vi "Configure Write LabVIEW Measurement File.vi"(0 "subVI":refnum<vi>, 2 "VI":refnum<vi>, 3 "ParentVI":refnum<vi>) -> (1 "Data Valid":bool)   [LabVIEW 2020]
doc: "Writes data to text-based measurement files (.lvm), binary measurement files (.tdm or .tdms), or Microsoft Excel files (.xlsx)."
uses:
  <vilib>/express/express shared/ExFile.llb/ex_FileFormats.ctl
  <vilib>/express/express shared/ExFile.llb/ex_userDefProperty.ctl
  <vilib>/express/express shared/ex_EditUserDefinedProperties/usiDataType.ctl
  <vilib>/express/express shared/ExFile.llb/ex_propertySource.ctl
  <vilib>/express/express output/ExFileWriteBlock.llb/ex_ExcelAdvancedConfig.ctl
  <vilib>/express/express shared/ExFile.llb/ex_FileGlobals.vi
  <vilib>/express/express shared/NI_ExcelFile/NI_ExcelFile.lvlib
panel:
  in  "timestamp":T1={"absolute time"=TRUE, "Timestamp format"=""}
  in  "Configure User Def Prop In":T5
  in  "Advanced":bool
  in  "Streaming":bool
  in  "always hostless warning":string="The current target will not have a host computer connected.  When you run this VI, it will return an error."
  in  "maybe hostless warning":string="The current target might not always have a host connected.  When you run this VI with no host connected, it will return an error."
  in  "delimiter":string
  in  "x_columns":enum32{"none", "one", "multiple"}(radio)
  in  "overwrite_mode":T6(radio)
  in  "column headings":enum32{"one per segment", "once", "none"}(radio)
  in  "delimiter enum":enum32{"tab", "comma"}(radio)
  in  "File path":path
  in  "Ask each iteration":bool
  in  "Ask only once":bool
  in  "Help":bool
  in  "Ok":bool
  in  "Cancel":bool
  in  "overwrite_mode_multi":i32
  in  "fixed_width":bool=TRUE
  in  "Width":i32=2 min=1 max=9
  in  "Samples":i32=1 min=1
  in  "Segments":i32=1 min=1
  in  "new_file_samples":bool
  in  "new_file_iter":bool
  in  "Time":i32 min=0 max=86399 format="%<%I:%M %p\n%m/%d/%y>T"
  in  "new_file_daily":bool
  in  "max_elapsed_seconds":i32 min=0 max=999
  in  "new_file_elaps_time":bool
  in  "KB":i32=100
  in  "new_file_size":bool=TRUE
  in  "Settings":bool
  in  "Save to series of files (multiple files)":bool
  in  "Save to one file":bool=TRUE
  in  "File Description":string
  in  "Ask user to choose file":bool
  in  "multi_file":bool
  in  "time_format_string":string="%Y-%m-%d"
  in  "new_file_mode":u16(ring)=2 items=["Date & Time", "Serial No.", "Both"]
  in  "Filename":path=path "test.lvm"
  in  "storage_format":T7
  # "Filename"
  # "File Format"
  # "Action"
  # "Segment Headers"
  # "X Value (Time) Columns"
  # "If a file already exists"
  # "Delimiter"
  # "File Description"
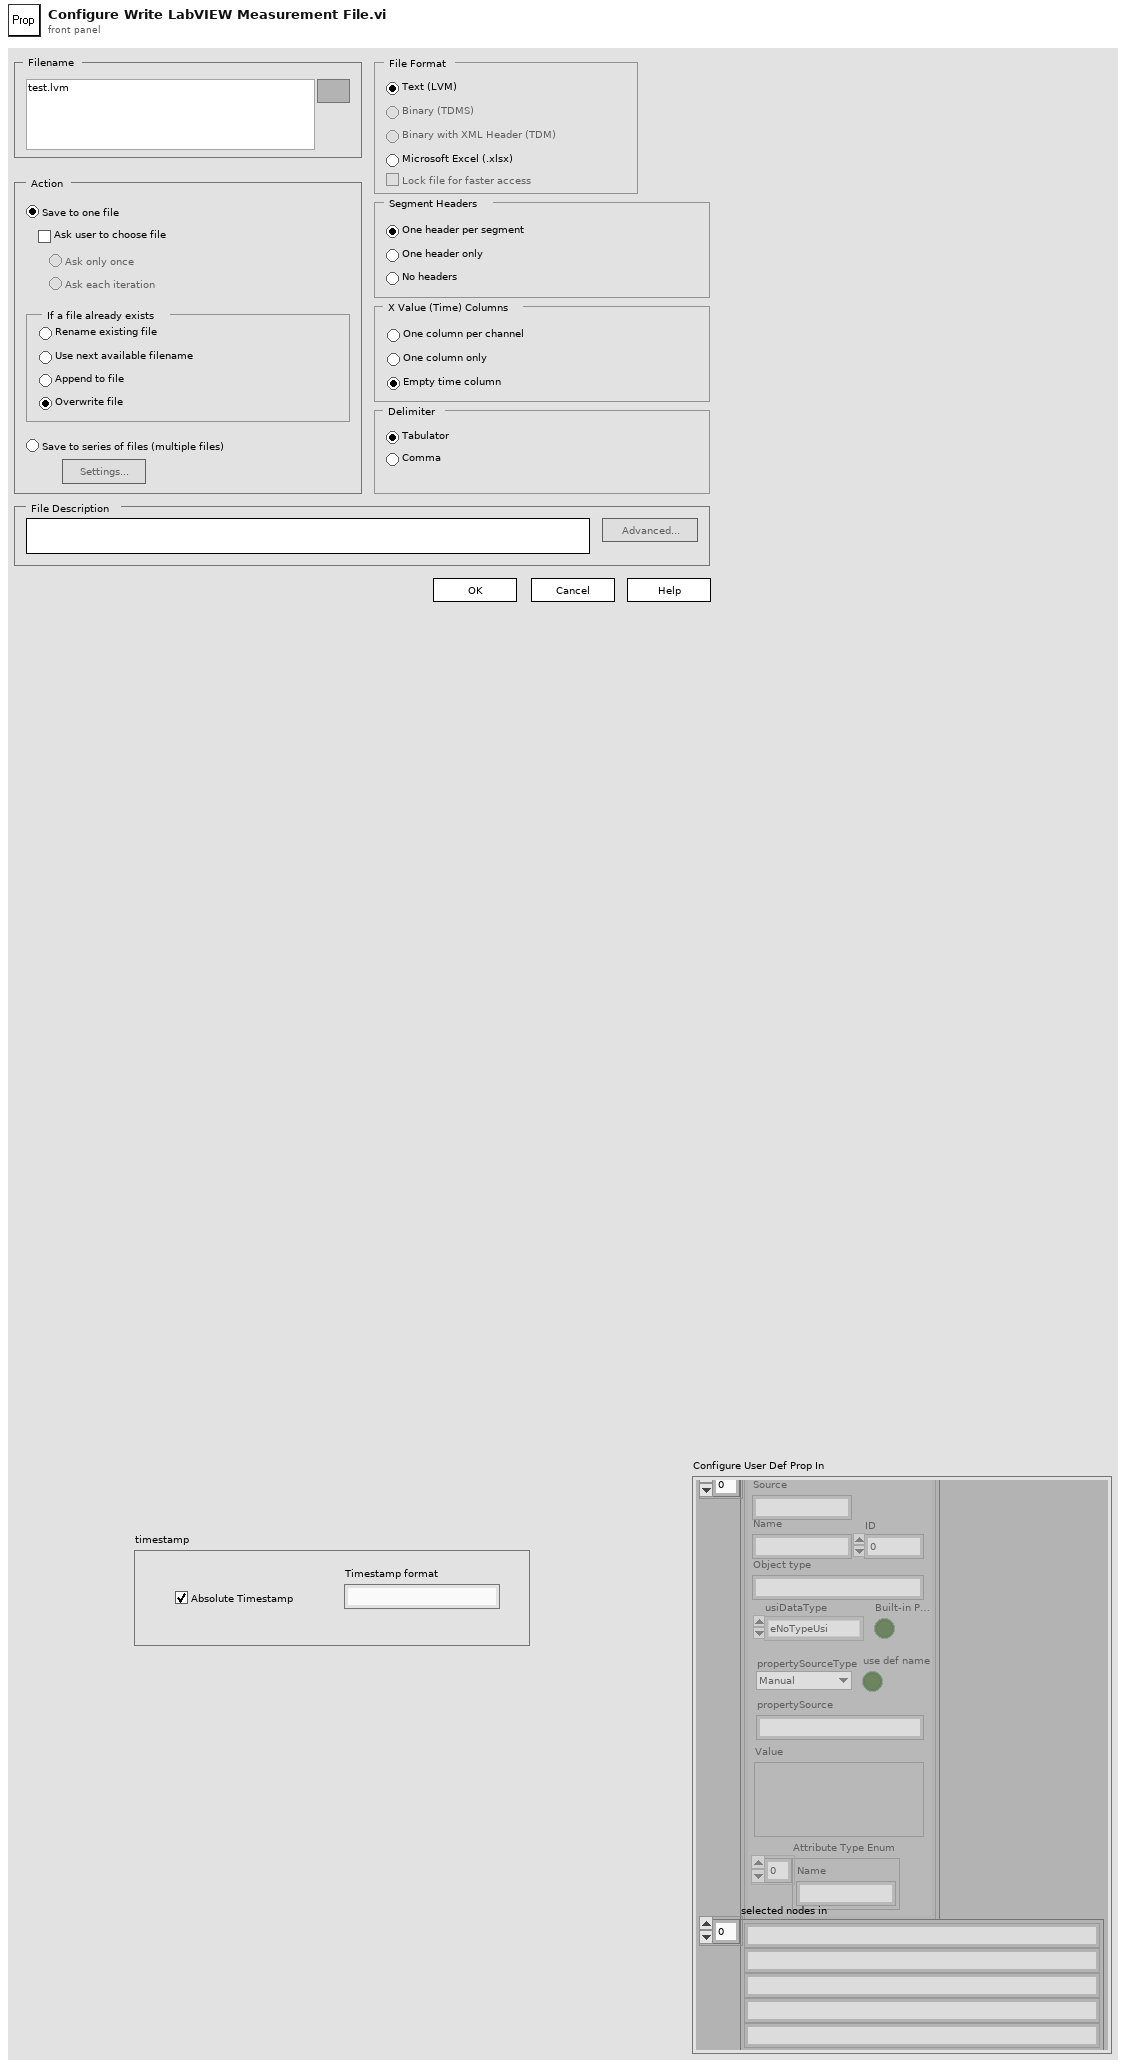
[diagram p1: front panel]
types:
  T1 = typedef "ex_ExcelAdvancedConfig.ctl" = cluster{"absolute time":bool, "Timestamp format":string}
  T2 = typedef "ex_userDefProperty.ctl" = cluster{"Name":string, "Object type":string, "usiDataType":T3, "propertySourceType":T4, "propertySource":string, "Value":variant, "ID":i32, "use def name":bool, "Source":string, "Built-in Prop":bool, "Attribute Type Enum":string[]}
  T3 = typedef "usiDataType.ctl" = enum16{"eNoTypeUsi", "eInt8Usi", "eInt16Usi", "eInt32Usi", "eInt64Usi", "eUInt8Usi", "eUInt16Usi", "eUInt32Usi", "eUInt64Usi", "eFloat32Usi", "eFloat64Usi", "- 0", "- 1", "- 2", "- 3", "- 4", "- 5", "- 6", "- 7", "- 8", "- 9", "eString8Usi", "eString16Usi", "eStringUsi", "eEnumUsi", "- 10", "- 11", "- 12", "- 13", "- 14", "eTimeUsi", "- 15", "- 16", "- 17", "- 18", "- 19", "- 20", "- 21", "- 22", "- 23", "eInstanceUsi", "eStoreUsi"}
  T4 = typedef "ex_propertySource.ctl" = enum16{"Manual", "System", "DAQmx Channel", "Terminal", "Ignore"}
  T5 = cluster{"user-def properties in":T2[], "selected nodes in":string[]}
  T6 = enum32{"overwrite", "overwrite & backup", "append", "next avail"}
  T7 = typedef "ex_FileFormats.ctl" = enum32{"lvm", "tdm", "tdms", "xlsx"}
  T8 = cluster{"Ctl Type":u16, "LV Express VI Ctl Label":string, "Wizard Ctl Label":string}[]
  T9 = typedef "propPageData.ctl" = cluster{"InstanceCtlRefs":refnum<vi>[], "ConfigDlgCtlRefs":refnum<vi>[], "Control Data":cluster{"Ctl Type":u16, "Instance Ctl Label":string, "Config Dialog Ctl Label":string}[], "viref Instance":refnum<vi>, "Types":i32[], "Config DialogVI":refnum<vi>}
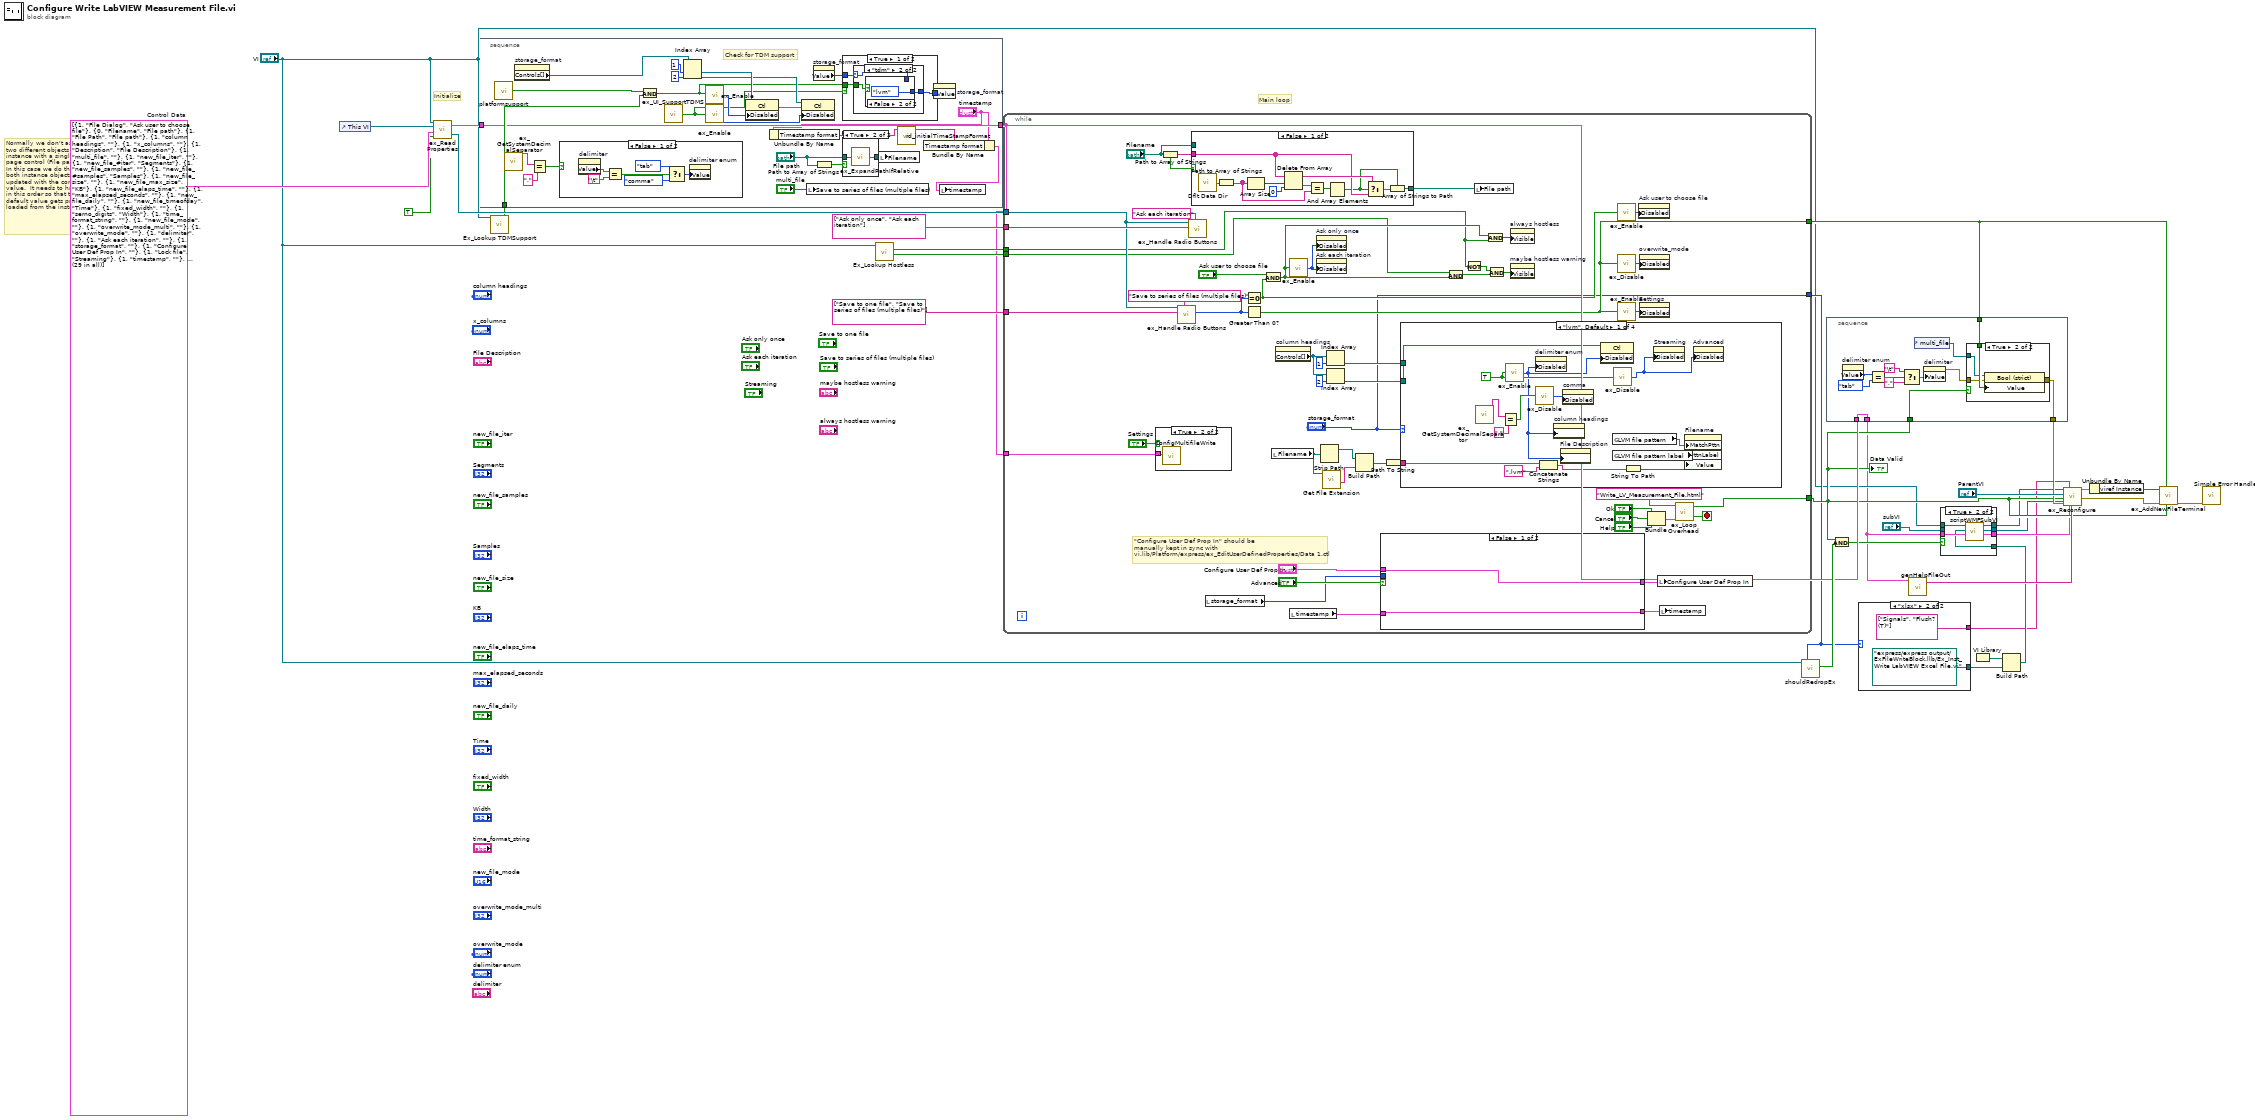
[diagram p0: block diagram]
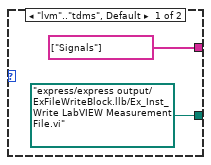
[diagram p3: hidden frame]
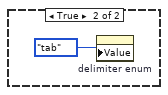
[diagram p5: hidden frame]
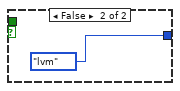
[diagram p8: hidden frame]
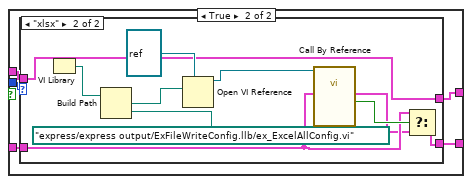
[diagram p10: hidden frame]
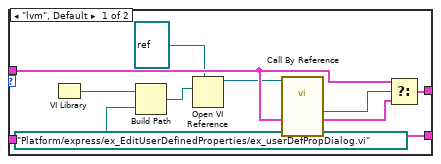
[diagram p11: hidden frame]
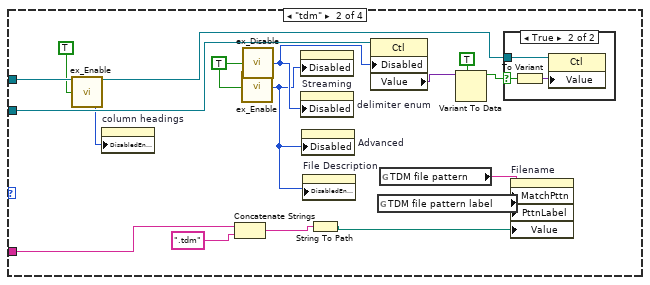
[diagram p12: hidden frame]
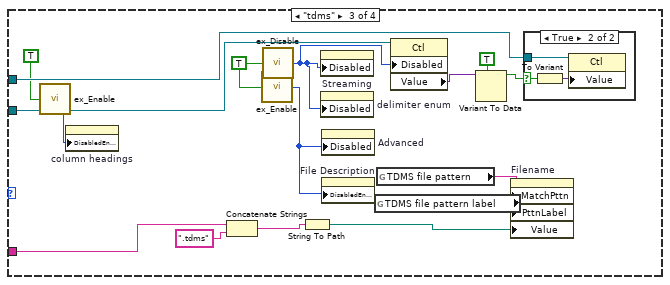
[diagram p14: hidden frame]
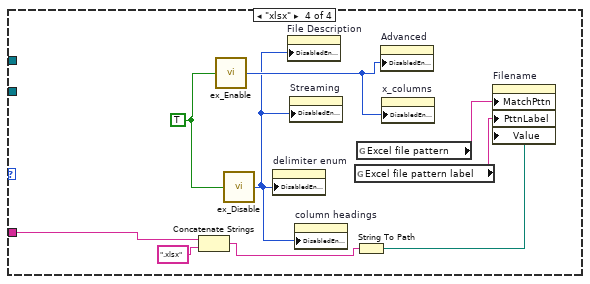
[diagram p16: hidden frame]
diagram:
  w25 = T8 [{"Ctl Type"=1, "LV Express VI Ctl Label"="File Dialog", "Wizard Ctl Label"="Ask user to choose file"}, {"Ctl Type"=0, "LV Express VI Ctl Label"="Filename", "Wizard Ctl Label"="File path"}, {"Ctl Type"=1, "LV Express VI Ctl Label"="File Path", "Wizard Ctl Label"="File path"}, {"Ctl Type"=1, "LV Express VI Ctl Label"="column headings", "Wizard Ctl Label"=""}, {"Ctl Type"=1, "LV Express VI Ctl Label"="x_columns", "Wizard Ctl Label"=""}, {"Ctl Type"=1, "LV Express VI Ctl Label"="Description", "Wizard Ctl Label"="File Description"}, {"Ctl Type"=1, "LV Express VI Ctl Label"="multi_file", "Wizard Ctl Label"=""}, {"Ctl Type"=1, "LV Express VI Ctl Label"="new_file_iter", "Wizard Ctl Label"=""}, {"Ctl Type"=1, "LV Express VI Ctl Label"="new_file_#iter", "Wizard Ctl Label"="Segments"}, {"Ctl Type"=1, "LV Express VI Ctl Label"="new_file_samples", "Wizard Ctl Label"=""}, {"Ctl Type"=1, "LV Express VI Ctl Label"="new_file_#samples", "Wizard Ctl Label"="Samples"}, {"Ctl Type"=1, "LV Express VI Ctl Label"="new_file_size", "Wizard Ctl Label"=""}, {"Ctl Type"=1, "LV Express VI Ctl Label"="new_file_max_size", "Wizard Ctl Label"="KB"}, {"Ctl Type"=1, "LV Express VI Ctl Label"="new_file_elaps_time", "Wizard Ctl Label"=""}, {"Ctl Type"=1, "LV Express VI Ctl Label"="max_elapsed_seconds", "Wizard Ctl Label"=""}, {"Ctl Type"=1, "LV Express VI Ctl Label"="new_file_daily", "Wizard Ctl Label"=""}, {"Ctl Type"=1, "LV Express VI Ctl Label"="new_file_timeofday", "Wizard Ctl Label"="Time"}, {"Ctl Type"=1, "LV Express VI Ctl Label"="fixed_width", "Wizard Ctl Label"=""}, {"Ctl Type"=1, "LV Express VI Ctl Label"="serno_digits", "Wizard Ctl Label"="Width"}, {"Ctl Type"=1, "LV Express VI Ctl Label"="time_format_string", "Wizard Ctl Label"=""}, {"Ctl Type"=1, "LV Express VI Ctl Label"="new_file_mode", "Wizard Ctl Label"=""}, {"Ctl Type"=1, "LV Express VI Ctl Label"="overwrite_mode_multi", "Wizard Ctl Label"=""}, {"Ctl Type"=1, "LV Express VI Ctl Label"="overwrite_mode", "Wizard Ctl Label"=""}, {"Ctl Type"=1, "LV Express VI Ctl Label"="delimiter", "Wizard Ctl Label"=""}, {"Ctl Type"=1, "LV Express VI Ctl Label"="Ask each iteration", "Wizard Ctl Label"=""}, {"Ctl Type"=1, "LV Express VI Ctl Label"="storage_format", "Wizard Ctl Label"=""}, {"Ctl Type"=1, "LV Express VI Ctl Label"="Configure User Def Prop In", "Wizard Ctl Label"=""}, {"Ctl Type"=1, "LV Express VI Ctl Label"="Lock file", "Wizard Ctl Label"="Streaming"}, {"Ctl Type"=1, "LV Express VI Ctl Label"="timestamp", "Wizard Ctl Label"=""}]  # Control Data
  # "Normally we don't associate\ntwo different objects on the\ninstance with a single config\npage control (File path).\nIn this case we do this so\nboth instance objects get\nupdated with the configured\nvalue.  It needs to happen\nin this order so that the\ndefault value gets properly\nloaded from the instance."
  # "Initialize"
  # "Main loop"
  n1 = control-ref of="This VI"() -> (w1:refnum<vi>)
  n2 = call <vilib>:"ex_Read Properties.vi"("Ignore Errors"=TRUE, "Control Data"=w25, "viref Configuration Dialog"=w1, "viref Instance"="VI") -> ("viref Configuration Dialog out"=w32:refnum<vi>, "Output Cluster"=w31:T9)  [unwired: 2 out]
  n3 = call <vilib>:"Ex_Lookup TDMSupport.vi"("VI RefNum for Context"="VI") -> ("TDM Support?"=w24:bool)  [unwired: 1 in, 9 out]
  n4 = stacked-sequence {
    tunnel: w31 -> [w36]
    tunnel: [w36] -> w17
    tunnel: w24 -> [w55]
    frame #0 {
      # "Check for TDM support"
      n5 = call <vilib>:"platformsupport.vi"() -> ("TDM Support for Platform"=w48:bool)  [unwired: 1 out]
      n6 = call <vilib>:"ex_GetSystemDecimalSeparator.vi"() -> ("Decimal Seperator"=w41:string)  [unwired: 11 out]
      n7 = property on="storage_format" class="RadioBtnsControl (strict)"() -> ("Controls[]"=w54:refnum<vi>[])  [unwired: 2 in, 2 out]
      n8 = Equal?(x=w41, y=",") -> (x = y?=w40:bool)
      n9 = case shown="False" w40 {
        frame False {
          n10 = property on="delimiter" class="Str"() -> ("Value"=w65:string)  [unwired: 2 in, 2 out]
          n11 = Equal?(x=w65, y="\t") -> (x = y?=w62:bool)
          n12 = Select(t=enum32{"tab", "comma"}."tab" ("delimiter enum"), s=w62, f=enum32{"tab", "comma"}."comma" ("delimiter enum")) -> (s? t:f=w61:enum32{"tab", "comma"})
          n13 = property on="delimiter enum" class="RadioBtnsControl (strict)"("Value"=w61) -> ()  [unwired: 2 in, 2 out]
        }
        frame True {
          n14 = property on="delimiter enum" class="RadioBtnsControl (strict)"("Value"=enum32{"tab", "comma"}."tab" ("delimiter enum")) -> ()  [unwired: 2 in, 2 out]
        }
      }
      n15 = And(x=w48, y=w55) -> (x .and. y?=w43:bool)
      n16 = call <vilib>:"ex_UI_SupportTDMS.vi"() -> ("support TDMSû"=w39:bool)  [unwired: 2 in]
      n17 = Index Array(array=w54, index #1=1, index #2=2 ("index")) -> (element #1=w53:refnum<vi>, element #2=w49:refnum<vi>)
      n18 = call <vilib>:"ex_Enable.vi"("Enable?"=w43) -> ("Disabled Value"=w45:u8)
      n19 = call <vilib>:"ex_Enable.vi"("Enable?"=w39) -> ("Disabled Value"=w47:u8)
      n20 = property class="Ctl"(reference=w53, "Disabled"=w45) -> (error out=w52:errorcluster)  [unwired: 1 in, 1 out]
      n21 = Unbundle By Name("timestamp") -> ("Timestamp format"=w34:string)
      n22 = property class="Ctl"(reference=w49, error in=w52, "Disabled"=w47) -> ()  [unwired: 2 out]
      n23 = local write "Save to series of files (multiple files)"("multi_file") -> ()
      n24 = property on="storage_format" class="RadioBtnsControl (strict)"() -> ("Value"=w46:T7)  [unwired: 2 in, 2 out]
      n25 = Path to Array of Strings(0:"File path") -> (1:w57:bool)  [unwired: 1 out]
      n26 = case shown="True" w57 {
        tunnel: "File path" -> [w77 w79]
        tunnel: [w77 w78] -> w59
        frame False {
        }
        frame True {
          n27 = call <vilib>:"ex_ExpandPathIfRelative.vi"("Path"=w79) -> ("Expanded path"=w78:path)  [unwired: 4 out]
        }
      }
      n28 = case shown="True" w39 {
        tunnel: w46 -> [w69 _]
        tunnel: w43 -> [w68 _]
        tunnel: [w67 enum32{"lvm", "tdm", "tdms"}."lvm"] -> w44
        frame True {
          n29 = case shown="\"tdm\"" w69 {
            selector: w69 -> [w70 w71]
            tunnel: w68 -> [_ w73]
            tunnel: [w70 w72] -> w67
            frame "lvm", Default {
            }
            frame "tdm" {
              n30 = case shown="False" w73 {
                tunnel: [w74 enum32{"lvm", "tdm", "tdms"}."lvm"] -> w72
                tunnel: w71 -> [w74 _]
                frame True {
                }
                frame False {
                }
              }
            }
          }
        }
        frame False {
        }
      }
      n31 = local write "Filename"(w59) -> ()
      n32 = call <vilib>:"rd_initialTimeStampFormat.vi"("timestamp format"=w34) -> ("timestamp format out"=w38:string)  [unwired: 9 in, 1 out]
      n33 = Bundle By Name(cluster="timestamp", "Timestamp format"=w38) -> (w37:T1)
      n34 = property on="storage_format" class="RadioBtnsControl (strict)"("Value"=w44) -> ()  [unwired: 2 in, 2 out]
      n35 = local write "timestamp"(w37) -> ()
    }
  }
  n36 = call <vilib>:"Ex_Lookup Hostless.vi"("VI RefNum for Context"="VI") -> ("Maybe Hostless"=w26:bool, "Always Hostless"=w27:bool)  [unwired: 1 in, 8 out]
  n37 = while {
    tunnel: [w128] -> w15
    tunnel: w32 -> [w113]
    tunnel: string[] ["Save to one file", "Save to series of files (multiple files)"] ("Radio Buttons") -> [w129]
    tunnel: w17 -> [w127]
    tunnel: string[] ["Ask only once", "Ask each iteration"] ("Radio Buttons") -> [w119]
    tunnel: [w106] -> w19
    tunnel: w27 -> [w95]
    tunnel: w26 -> [w94]
    tunnel: ["storage_format"] -> w13
    stop <- w126 stop-if-true
    # "\"Configure User Def Prop In\" should be\nmanually kept in sync with \nvi.lib/Platform/express/ex_EditUserDefinedProperties/Data 1.ctl"
    n38 = case shown="True" "Settings" {
      tunnel: w127 -> [_ w230]
      frame False {
      }
      frame True {
        n39 = call <vilib>:"ConfigMultifileWrite.vi"("Reference"=w230) -> ()  [unwired: 11 out]
      }
    }
    n40 = Path to Array of Strings(0:"Filename") -> (1:w116:bool, 2:w117:string[])
    n41 = call <vilib>:"ex_Handle Radio Buttons.vi"("Boolean Control"="Save to series of files (multiple files)" ("Numeric Control"), "Radio Buttons"=w129, "VI refnum"=w113) -> ("Selected Button"=w104:u32)  [unwired: 4 in, 4 out]
    n42 = call <vilib>:"ex_Handle Radio Buttons.vi"("Boolean Control"="Ask each iteration" ("Numeric Control"), "Radio Buttons"=w119, "VI refnum"=w113) -> ()  [unwired: 4 in, 5 out]
    n43 = case shown="False" w116 {
      tunnel: [w220 w229] -> w115
      tunnel: "Filename" -> [_ w229]
      tunnel: w117 -> [w219 _]
      frame False {
        n44 = call <vilib>:"Dflt Data Dir.vi"() -> ("App:Default Data Directory"=w221:path)
        n45 = Path to Array of Strings(0:w221) -> (2:w228:string[])  [unwired: 1 out]
        n46 = Array Size(array=w228) -> (size(s)=w222:i32)
        n47 = Delete From Array(array=w219, length=w222, index=0) -> (deleted portion=w227:string[], array with subset deleted=w226:string[])
        n48 = Equal?(x=w227, y=w228) -> (x = y?=w224:bool[])
        n49 = And Array Elements(Boolean array=w224) -> (logical AND=w218:bool)
        n50 = Select(t=w226, s=w218, f=w219) -> (s? t:f=w225:string[])
        n51 = Array of Strings to Path(0:w225, 1:w218) -> (2:w220:path)
      }
      frame True {
      }
    }
    n52 = local read "storage_format"() -> (w83:T7)
    n53 = Equal To 0?(x=w104) -> (x = 0?=w102:bool)
    n54 = Greater Than 0?(x=w104) -> (x > 0?=w106:bool)
    n55 = And(x="Ask user to choose file", y=w102) -> (x .and. y?=w96:bool)
    n56 = local read "Filename"() -> (w88:path)
    n57 = property on="column headings" class="RadioBtnsControl (strict)"() -> ("Controls[]"=w109:refnum<vi>[])  [unwired: 2 in, 2 out]
    n58 = call <vilib>:"ex_Enable.vi"("Enable?"=w96) -> ("Disabled Value"=w120:u8)
    n59 = local read "timestamp"() -> (w80:T1)
    n60 = property on="Ask only once" class="Bool (strict)"("Disabled"=w120) -> ()  [unwired: 2 in, 2 out]
    n61 = property on="Ask each iteration" class="Bool (strict)"("Disabled"=w120) -> ()  [unwired: 2 in, 2 out]
    n62 = Strip Path(path=w88) -> (stripped path=w87:path)  [unwired: 1 out]
    n63 = call <vilib>:"Get File Extension.vi"("file"=w88) -> ("filename without extension"=w86:string)  [unwired: 1 in, 9 out]
    n64 = Index Array(array=w109, index=1) -> (element=w107:refnum<vi>)
    n65 = Index Array(array=w109, index=2) -> (element=w110:refnum<vi>)
    n66 = Build Path(base path=w87, name or relative path=w86) -> (appended path=w85:path)
    n67 = case shown="False" "Advanced" {
      tunnel: [w131 w136] -> w93
      tunnel: "Configure User Def Prop In" -> [w131 w135]
      tunnel: w83 -> [_ w134]
      tunnel: w80 -> [w130 w133]
      tunnel: [w130 w132] -> w82
      frame False {
      }
      frame True {
        n68 = case shown="\"xlsx\"" w134 {
          tunnel: [w146 w147] -> w136
          tunnel: w135 -> [w145 w147]
          tunnel: w133 -> [w137 w150]
          tunnel: [w137 w148] -> w132
          frame "lvm", Default {
            n69 = VI Library() -> (path=w140:path)
            n70 = Build Path(base path=w140, name or relative path=path "Platform/express/ex_EditUserDefinedProperties/ex_userDefPropDialog.vi") -> (appended path=w141:path)
            n71 = Open VI Reference(type specifier VI Refnum (for type only)=refnum<vi> refnum, vi path=w141) -> (vi reference=w139:refnum<vi>)  [unwired: 1 in, 4 out]
            n72 = call-by-ref "?"(reference=w139, "Configure User Def Prop Control"=w145) -> ("Data Out"=w143:T5, "Cancelled?"=w144:bool)  [unwired: 10 in, 2 out]
            n73 = Select(t=w145, s=w144, f=w143) -> (s? t:f=w146:T5)
          }
          frame "xlsx" {
            n74 = VI Library() -> (path=w156:path)
            n75 = Build Path(base path=w156, name or relative path=path "express/express output/ExFileWriteConfig.llb/ex_ExcelAllConfig.vi") -> (appended path=w154:path)
            n76 = Open VI Reference(type specifier VI Refnum (for type only)=refnum<vi> refnum, vi path=w154) -> (vi reference=w153:refnum<vi>)  [unwired: 4 in, 1 out]
            n77 = call-by-ref "?"(reference=w153, "timestamp input"=w150) -> ("Cancel?"=w151:bool, "timestamp output"=w149:T1)  [unwired: 10 in, 2 out]
            n78 = Select(t=w150, s=w151, f=w149) -> (s? t:f=w148:T1)
          }
        }
      }
    }
    n79 = Path To String(path=w85) -> (string=w84:string)
    n80 = case shown="\"lvm\", Default" "storage_format" {
      tunnel: w110 -> [w170 w186 w205 _]
      tunnel: w107 -> [_ w185 w204 _]
      tunnel: w84 -> [w162 w179 w200 w213]
      frame "lvm", Default {
        w167 = TRUE ("Enable?")
        n81 = call <vilib>:"ex_GetSystemDecimalSeparator.vi"() -> ("Decimal Seperator"=w159:string)  [unwired: 11 out]
        n82 = Equal?(x=w159, y=",") -> (x = y?=w158:bool)
        n83 = call <vilib>:"ex_Enable.vi"("Enable?"=w167) -> ("Disabled Value"=w157:u8)
        n84 = property on="delimiter enum" class="RadioBtnsControl (strict)"("Disabled"=w157) -> ()  [unwired: 2 in, 2 out]
        n85 = call <vilib>:"ex_Disable.vi"("Disable?"=w158) -> ("Disabled value"=w160:u8)
        n86 = Concatenate Strings(w162, ".lvm" ("replace string (\"\")")) -> (w164:string)
        n87 = property on="column headings" class="RadioBtnsControl (strict)"("DisabledEnum"=w157) -> ()  [unwired: 2 in, 2 out]
        n88 = property on="File Description" class="Str"("DisabledEnum"=w157) -> ()  [unwired: 2 in, 2 out]
        n89 = property on="comma" class="Bool (strict)"("Disabled"=w160) -> ()  [unwired: 2 in, 2 out]
        n90 = property class="Ctl"(reference=w170, "Disabled"=w157) -> ()  [unwired: 1 in, 2 out]
        n91 = global read "ex_FileGlobals.vi" "LVM file pattern"() -> (w169:string)
        n92 = global read "ex_FileGlobals.vi" "LVM file pattern label"() -> (w168:string)
        n93 = call <vilib>:"ex_Disable.vi"("Disable?"=w167) -> ("Disabled value"=w166:u8)
        n94 = String To Path(string=w164) -> (path=w163:path)
        n95 = property on="Streaming" class="Bool (strict)"("Disabled"=w166) -> ()  [unwired: 2 in, 2 out]
        n96 = property on="Filename" class="Path"("MatchPttn"=w169, "PttnLabel"=w168, "Value"=w163) -> ()  [unwired: 2 in, 2 out]
        n97 = property on="Advanced" class="Bool"("Disabled"=w166) -> ()  [unwired: 2 in, 2 out]
      }
      frame "tdm" {
        w173 = TRUE ("Disable?")
        n98 = call <vilib>:"ex_Enable.vi"("Enable?"=TRUE ("Disable?")) -> ("Disabled Value"=w177:u8)
        n99 = property on="column headings" class="RadioBtnsControl (strict)"("DisabledEnum"=w177) -> ()  [unwired: 2 in, 2 out]
        n100 = Concatenate Strings(w179, ".tdm" ("replace string (\"\")")) -> (w181:string)
        n101 = call <vilib>:"ex_Enable.vi"("Enable?"=w173) -> ("Disabled Value"=w171:u8)
        n102 = call <vilib>:"ex_Disable.vi"("Disable?"=w173) -> ("Disabled value"=w172:u8)
        n103 = property on="Streaming" class="Bool (strict)"("Disabled"=w171) -> ()  [unwired: 2 in, 2 out]
        n104 = property on="delimiter enum" class="RadioBtnsControl (strict)"("Disabled"=w172) -> ()  [unwired: 2 in, 2 out]
        n105 = property on="Advanced" class="Bool"("Disabled"=w171) -> ()  [unwired: 2 in, 2 out]
        n106 = property on="File Description" class="Str"("DisabledEnum"=w171) -> ()  [unwired: 2 in, 2 out]
        n107 = String To Path(string=w181) -> (path=w180:path)
        n108 = property class="Ctl"(reference=w186, "Disabled"=w172) -> ("Value"=w176:variant)  [unwired: 1 in, 2 out]
        n109 = global read "ex_FileGlobals.vi" "TDM file pattern label"() -> (w183:string)
        n110 = global read "ex_FileGlobals.vi" "TDM file pattern"() -> (w184:string)
        n111 = Variant To Data(type=TRUE, Variant=w176) -> (data=w174:bool)  [unwired: 1 in, 1 out]
        n112 = case shown="True" w174 {
          selector: w174 -> [_ w188]
          tunnel: w185 -> [_ w189]
          frame False {
          }
          frame True {
            n113 = To Variant(anything=w188) -> (Variant=w187:variant)
            n114 = property class="Ctl"(reference=w189, "Value"=w187) -> ()  [unwired: 1 in, 2 out]
          }
        }
        n115 = property on="Filename" class="Path"("MatchPttn"=w184, "PttnLabel"=w183, "Value"=w180) -> ()  [unwired: 2 in, 2 out]
      }
      frame "tdms" {
        w192 = TRUE ("Disable?")
        n116 = call <vilib>:"ex_Enable.vi"("Enable?"=TRUE ("Disable?")) -> ("Disabled Value"=w196:u8)
        n117 = property on="column headings" class="RadioBtnsControl (strict)"("DisabledEnum"=w196) -> ()  [unwired: 2 in, 2 out]
        n118 = Concatenate Strings(w200, ".tdms" ("replace string (\"\")")) -> (w198:string)
        n119 = call <vilib>:"ex_Enable.vi"("Enable?"=w192) -> ("Disabled Value"=w190:u8)
        n120 = call <vilib>:"ex_Disable.vi"("Disable?"=w192) -> ("Disabled value"=w191:u8)
        n121 = String To Path(string=w198) -> (path=w203:path)
        n122 = property on="Streaming" class="Bool (strict)"("Disabled"=w191) -> ()  [unwired: 2 in, 2 out]
        n123 = property on="delimiter enum" class="RadioBtnsControl (strict)"("Disabled"=w191) -> ()  [unwired: 2 in, 2 out]
        n124 = property on="Advanced" class="Bool"("Disabled"=w190) -> ()  [unwired: 2 in, 2 out]
        n125 = property on="File Description" class="Str"("DisabledEnum"=w190) -> ()  [unwired: 2 in, 2 out]
        n126 = global read "ex_FileGlobals.vi" "TDMS file pattern label"() -> (w201:string)
        n127 = global read "ex_FileGlobals.vi" "TDMS file pattern"() -> (w202:string)
        n128 = property class="Ctl"(reference=w205, "Disabled"=w191) -> ("Value"=w195:variant)  [unwired: 1 in, 2 out]
        n129 = Variant To Data(type=TRUE, Variant=w195) -> (data=w193:bool)  [unwired: 1 in, 1 out]
        n130 = property on="Filename" class="Path"("MatchPttn"=w202, "PttnLabel"=w201, "Value"=w203) -> ()  [unwired: 2 in, 2 out]
        n131 = case shown="True" w193 {
          selector: w193 -> [_ w207]
          tunnel: w204 -> [_ w208]
          frame False {
          }
          frame True {
            n132 = To Variant(anything=w207) -> (Variant=w206:variant)
            n133 = property class="Ctl"(reference=w208, "Value"=w206) -> ()  [unwired: 1 in, 2 out]
          }
        }
      }
      frame "xlsx" {
        w216 = TRUE
        n134 = Concatenate Strings(w213, ".xlsx" ("string")) -> (w211:string)
        n135 = call <vilib>:"ex_Enable.vi"("Enable?"=w216) -> ("Disabled Value"=w217:u8)
        n136 = call <vilib>:"ex_Disable.vi"("Disable?"=w216) -> ("Disabled value"=w209:u8)
        n137 = property on="delimiter enum" class="RadioBtnsControl (strict)"("DisabledEnum"=w209) -> ()  [unwired: 2 in, 2 out]
        n138 = property on="File Description" class="Str"("DisabledEnum"=w209) -> ()  [unwired: 2 in, 2 out]
        n139 = property on="Streaming" class="Bool (strict)"("DisabledEnum"=w209) -> ()  [unwired: 2 in, 2 out]
        n140 = property on="column headings" class="RadioBtnsControl (strict)"("DisabledEnum"=w209) -> ()  [unwired: 2 in, 2 out]
        n141 = global read "ex_FileGlobals.vi" "Excel file pattern label"() -> (w214:string)
        n142 = String To Path(string=w211) -> (path=w210:path)
        n143 = global read "ex_FileGlobals.vi" "Excel file pattern"() -> (w215:string)
        n144 = property on="Advanced" class="Bool"("DisabledEnum"=w217) -> ()  [unwired: 2 in, 2 out]
        n145 = property on="x_columns" class="RadioBtnsControl (strict)"("DisabledEnum"=w217) -> ()  [unwired: 2 in, 2 out]
        n146 = property on="Filename" class="Path"("MatchPttn"=w215, "PttnLabel"=w214, "Value"=w210) -> ()  [unwired: 2 in, 2 out]
      }
    }
    n147 = And(x=w94, y=w96) -> (x .and. y?=w101:bool)
    n148 = Not(x=w95) -> (.not. x?=w100:bool)
    n149 = local write "File path"(w115) -> ()
    n150 = And(x=w96, y=w95) -> (x .and. y?=w98:bool)
    n151 = And(x=w100, y=w101) -> (x .and. y?=w99:bool)
    n152 = property on="always hostless" class="Str"("Visible"=w98) -> ()  [unwired: 2 in, 2 out]
    n153 = property on="maybe hostless warning" class="Str"("Visible"=w99) -> ()  [unwired: 2 in, 2 out]
    n154 = call <vilib>:"ex_Enable.vi"("Enable?"=w102) -> ("Disabled Value"=w103:u8)
    n155 = call <vilib>:"ex_Disable.vi"("Disable?"=w106) -> ("Disabled value"=w112:u8)
    n156 = call <vilib>:"ex_Enable.vi"("Enable?"=w106) -> ("Disabled Value"=w105:u8)
    n157 = property on="Ask user to choose file" class="Bool (strict)"("Disabled"=w103) -> ()  [unwired: 2 in, 2 out]
    n158 = property on="overwrite_mode" class="RadioBtnsControl (strict)"("Disabled"=w112) -> ()  [unwired: 2 in, 2 out]
    n159 = property on="Settings" class="Bool"("Disabled"=w105) -> ()  [unwired: 2 in, 2 out]
    n160 = Bundle("Ok"="Ok", "Cancel"="Cancel", "Help"="Help") -> (w121:cluster{"Ok":bool, "Cancel":bool, "Help":bool})  [unwired: 1 out]
    n161 = local write "Configure User Def Prop In"(w93) -> ()
    n162 = local write "timestamp"(w82) -> ()
    n163 = call <vilib>:"ex_Loop Overhead.vi"("Bottom Button Bar"=w121, "Help string to search for"="Write_LV_Measurement_File.html") -> ("Loop Terminator"=w126:bool, "Data Valid"=w128:bool)  [unwired: 1 in, 1 out]
  }
  "Data Valid" <- w15
  n164 = call <vilib>:"shouldRedropEx.vi"("storage_format"=w13, "VI"="VI") -> ("redrop?"=w21:bool)  [unwired: 9 in]
  n165 = stacked-sequence {
    tunnel: w19 -> [w236]
    tunnel: w15 -> [w235]
    tunnel: [w232] -> w18
    tunnel: w17 -> [w231]
    tunnel: [w231] -> w9
    frame #0 {
      n166 = property on="delimiter enum" class="RadioBtnsControl (strict)"() -> ("Value"=w241:enum32{"tab", "comma"})  [unwired: 2 in, 2 out]
      n167 = Equal?(x=w241, y=enum32{"tab", "comma"}."tab" ("delimiter enum")) -> (x = y?=w242:bool)
      n168 = Select(t="\t", s=w242, f=",") -> (s? t:f=w237:string)
      n169 = control-ref of="multi_file"() -> (w234:refnum<vi>)
      n170 = property on="delimiter" class="Str"("Value"=w237) -> (error out=w233:errorcluster)  [unwired: 2 in, 1 out]
      n171 = case shown="True" w235 {
        tunnel: w236 -> [_ w247]
        tunnel: w234 -> [_ w246]
        tunnel: w233 -> [w243 w245]
        tunnel: [w243 w244] -> w232
        frame False {
        }
        frame True {
          n172 = property class="Bool (strict)"(reference=w246, error in=w245, "Value"=w247) -> (error out=w244:errorcluster)  [unwired: 1 out]
        }
      }
    }
  }
  n173 = And(x=w15, y=w21) -> (x .and. y?=w12:bool)
  n174 = case shown="\"xlsx\"" w13 {
    tunnel: [path "express/express output/ExFileWriteBlock.llb/Ex_Inst_Write LabVIEW Measurement File.vi" ("path") path "express/express output/ExFileWriteBlock.llb/Ex_Inst_Write LabVIEW Excel File.vi" ("path")] -> w4
    tunnel: [string[] ["Signals"] ("Inputs/Outputs to Grow") string[] ["Signals", "Flush? (T)"] ("Inputs/Outputs to Grow")] -> w2
    frame "lvm".."tdms", Default {
    }
    frame "xlsx" {
    }
  }
  n175 = call <vilib>:"genHelpFileOut.vi"("Output Cluster"=w9) -> ("Help Description"=w30:string)  [unwired: 5 out]
  n176 = VI Library() -> (path=w5:path)
  n177 = Build Path(base path=w5, name or relative path=w4) -> (appended path=w3:path)
  n178 = case shown="True" w12 {
    tunnel: "VI" -> [w254 _]
    tunnel: [w254 w260] -> w8
    tunnel: [w253 w259] -> w7
    tunnel: [w252 w258] -> w6
    tunnel: "subVI" -> [w253 w257]
    tunnel: w9 -> [w252 w256]
    tunnel: w3 -> [_ w255]
    frame False {
    }
    frame True {
      n179 = call <vilib>:"scriptWMFSubVI.vi"("props cluster"=w256, "path"=w255, "subVI in"=w257) -> ("props cluster out"=w258:T9, "subVI out"=w259:refnum<vi>, "VI out"=w260:refnum<vi>)  [unwired: 5 in, 1 out]
    }
  }
  n180 = call <vilib>:"ex_Reconfigure.vi"("VI refnum"=w8, "Parent VI refnum"="ParentVI", "Data Valid"=w15, "subVI refnum"=w7, "error in"=w18, "Inputs/Outputs to Grow"=w2, "Props Cluster"=w6, "Configuration Description"=w30) -> ("Props Cluster Out"=w20:T9, "error out"=w22:errorcluster)  [unwired: 5 in, 13 out]
  n181 = Unbundle By Name(w20) -> ("viref Instance"=w16:refnum<vi>)
  n182 = call <vilib>:"ex_AddNewFileTerminal.vi"("Data Valid"=w15, "Boolean"=w19, "error in"=w22, "VI"=w16) -> ("error out"=w14:errorcluster)  [unwired: 1 in, 6 out]
  n183 = call <vilib>:"Simple Error Handler.vi"("error in (no error)"=w14) -> ()  [unwired: 1 in, 8 out]
